vi "PythonToLabview.vi"() -> ()   [LabVIEW 2019]
panel:
  out "Input-PORT":u16
  in  "FIX DONE":bool
  out "ALLAM":bool
  out "Resuilt":string
  out "Confidence":dbl(slide) scale=0.0..1.0
  out "Target_bin":string
  out "Color_detected":string
  out "Status":string
  out "Timestamp":timestamp format="%<%Y-%m-%d_%H:%M:%S>T"
  out "Robot_id":string
  in  "OPERATE":bool
  in  "STATUS":bool
  in  "ERRO-CODE":u16
  in  "DECISION":u16(slide) scale=1.0..4.0
  out "data-in":string
  # "Notes:\n- STATUS: Power on/off\n-  OPERATE: Arm state\n- DECISION: Branch selection\n- ERROR-CODE: Error code (\"0\" mean no error)"
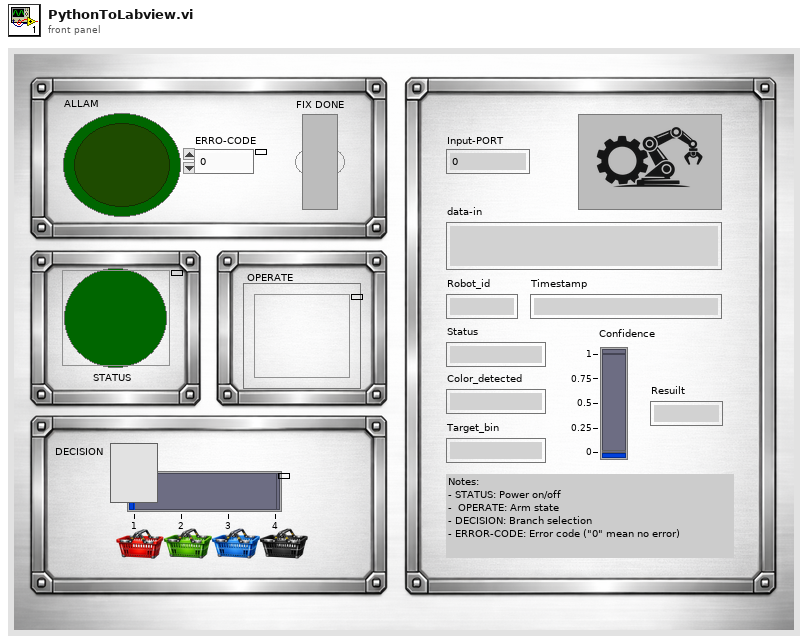
[diagram p1: front panel]
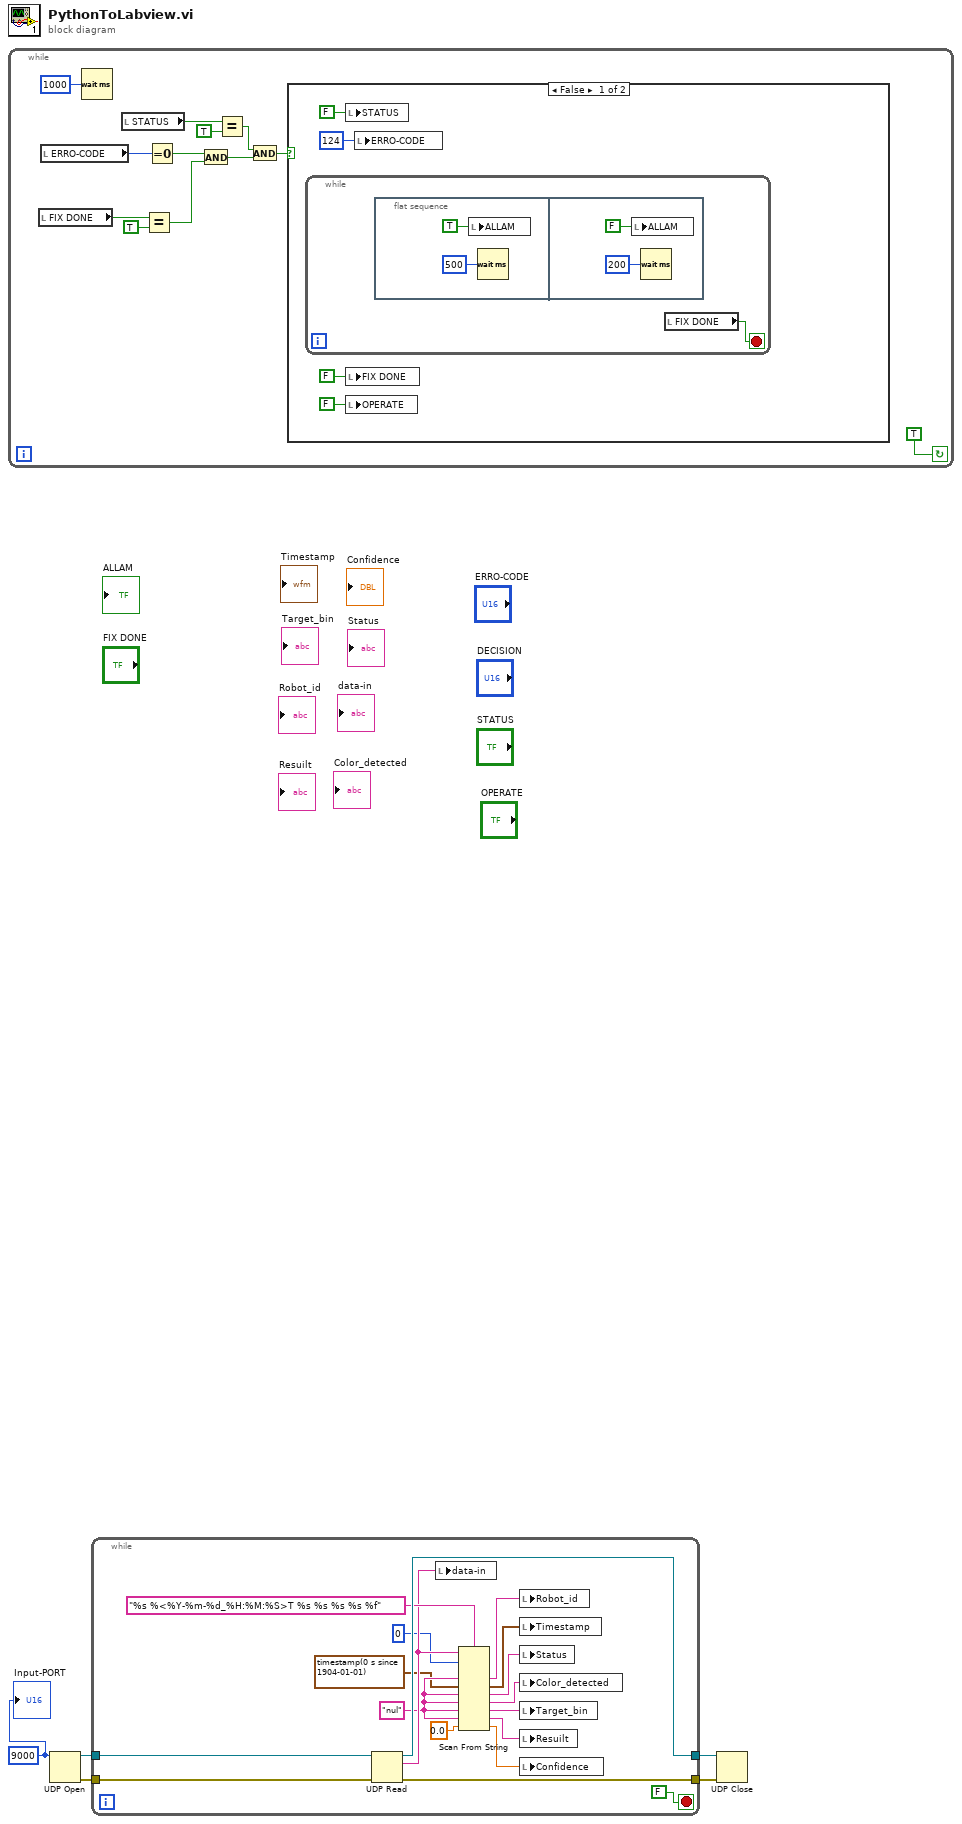
[diagram p0: block diagram]
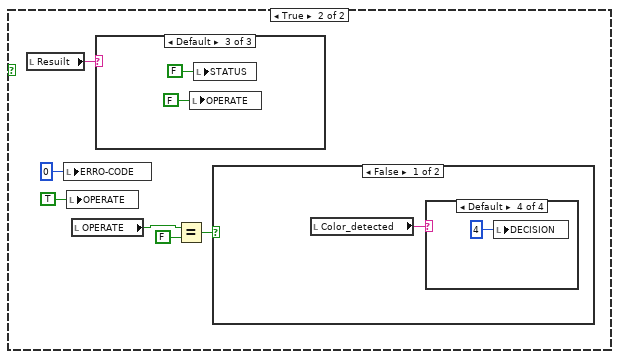
[diagram p2: hidden frame]
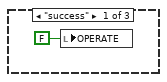
[diagram p3: hidden frame]
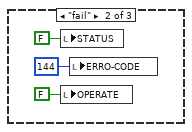
[diagram p4: hidden frame]
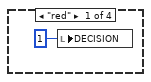
[diagram p5: hidden frame]
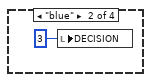
[diagram p6: hidden frame]
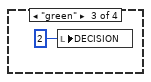
[diagram p7: hidden frame]
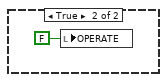
[diagram p8: hidden frame]
diagram:
  w1 = u16 9000 ("port")
  n1 = while {
    stop <- TRUE ("y") continue-if-true
    n2 = local read "FIX DONE"() -> (w10:bool)
    n3 = local read "ERRO-CODE"() -> (w16:u16)
    n4 = Wait (ms)(milliseconds to wait=u32 1000) -> ()  [unwired: 1 out]
    n5 = local read "STATUS"() -> (w14:bool)
    n6 = Equal?(x=w10, y=TRUE) -> (x = y?=w8:bool)
    n7 = Equal To 0?(x=w16) -> (x = 0?=w7:bool)
    n8 = And(x=w7, y=w8) -> (x .and. y?=w11:bool)
    n9 = Equal?(x=w14, y=TRUE) -> (x = y?=w15:bool)
    n10 = And(x=w15, y=w11) -> (x .and. y?=w17:bool)
    n11 = case shown="False" w17 {
      frame False {
        n12 = while {
          stop <- w22 stop-if-true
          n13 = flat-sequence {
            frame #0 {
              n14 = local write "ALLAM"(TRUE ("ALAM")) -> ()
              n15 = Wait (ms)(milliseconds to wait=u32 500) -> ()  [unwired: 1 out]
            }
            frame #1 {
              n16 = local write "ALLAM"(FALSE ("ALAM")) -> ()
              n17 = Wait (ms)(milliseconds to wait=u32 200) -> ()  [unwired: 1 out]
            }
          }
          n18 = local read "FIX DONE"() -> (w22:bool)
        }
        n19 = local write "STATUS"(FALSE ("M2")) -> ()
        n20 = local write "FIX DONE"(FALSE ("FIX DONE")) -> ()
        n21 = local write "OPERATE"(FALSE ("M1")) -> ()
        n22 = local write "ERRO-CODE"(u16 124 ("D2")) -> ()
      }
      frame True {
        n23 = local read "Resuilt"() -> (w28:string)
        n24 = local write "ERRO-CODE"(u16 0 ("D2")) -> ()
        n25 = local write "OPERATE"(TRUE ("M1")) -> ()
        n26 = local read "OPERATE"() -> (w31:bool)
        n27 = case shown="Default" w28 {
          frame "success" {
            n28 = local write "OPERATE"(FALSE ("M1")) -> ()
          }
          frame "fail" {
            n29 = local write "STATUS"(FALSE ("M2")) -> ()
            n30 = local write "OPERATE"(FALSE ("M1")) -> ()
            n31 = local write "ERRO-CODE"(u16 144 ("D2")) -> ()
          }
          frame Default {
            n32 = local write "OPERATE"(FALSE ("M1")) -> ()
            n33 = local write "STATUS"(FALSE ("M2")) -> ()
          }
        }
        n34 = Equal?(x=w31, y=FALSE) -> (x = y?=w29:bool)
        n35 = case shown="False" w29 {
          frame False {
            n36 = local read "Color_detected"() -> (w39:string)
            n37 = case shown="Default" w39 {
              frame "red" {
                n38 = local write "DECISION"(u16 1 ("D1")) -> ()
              }
              frame "blue" {
                n39 = local write "DECISION"(u16 3 ("D1")) -> ()
              }
              frame "green" {
                n40 = local write "DECISION"(u16 2 ("D1")) -> ()
              }
              frame Default {
                n41 = local write "DECISION"(u16 4 ("D1")) -> ()
              }
            }
          }
          frame True {
            n42 = local write "OPERATE"(FALSE ("M1")) -> ()
          }
        }
      }
    }
  }
  n43 = UDP Open(11:w1) -> (port=w5:refnum<k16>, 0:w2:errorcluster)  [unwired: 4 in, 1 out]
  n44 = while {
    tunnel: w5 -> [w62]
    tunnel: [w61] -> w4
    tunnel: [w57] -> w3
    tunnel: w2 -> [w56]
    stop <- FALSE stop-if-true
    w47 = "nul" ("default value 1")
    n45 = UDP Read(connection ID=w62, 8:w56) -> (data out=w59:string, error out=w57:errorcluster, 3:w61:refnum<k16>)  [unwired: 2 in, 2 out]
    n46 = local write "data-in"(w59) -> ()
    n47 = Scan From String(format string="%s %<%Y-%m-%d_%H:%M:%S>T %s %s %s %s %f", input string=w59, initial scan location=u32 0, default 1=w47, default 2=timestamp(0 s since 1904-01-01) ("default value 2"), default 3=w47, default 4=w47, default 5=w47, default 6=w47, default 7=0.0 ("default value 7")) -> (output 1=w54:string, output 2=w53:timestamp, output 3=w52:string, output 4=w51:string, output 5=w50:string, output 6=w49:string, output 7=w48:dbl)  [unwired: 1 in, 3 out]
    n48 = local write "Robot_id"(w54) -> ()
    n49 = local write "Timestamp"(w53) -> ()
    n50 = local write "Status"(w52) -> ()
    n51 = local write "Color_detected"(w51) -> ()
    n52 = local write "Target_bin"(w50) -> ()
    n53 = local write "Resuilt"(w49) -> ()
    n54 = local write "Confidence"(w48) -> ()
  }
  n55 = UDP Close(connection ID=w4, 8:w3) -> ()  [unwired: 2 out]
  "Input-PORT" <- w1
